vi "Dequeue.vi"(8 "error in (no error)":errorcluster, 10 "Dequeue Mode":T1, 11 "Messaging in":refnum<class "Messaging.lvclass">) -> (0 "error out":errorcluster, 1 "Data":variant, 2 "Message":string, 3 "Messaging out":refnum<class "Messaging.lvclass">)   [LabVIEW 2023, in "Messaging.lvclass"]
uses:
  Messaging.lvclass
  Messaging.lvclass/Messaging.ctl
  Msg/Msg.Q.DequeueMode.ctl
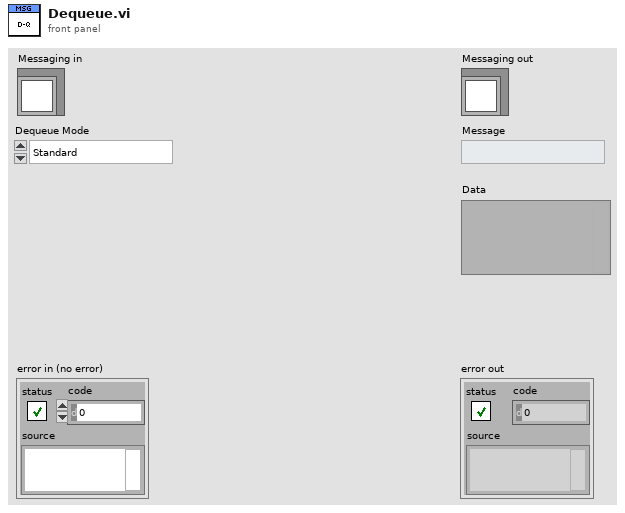
[diagram p1: front panel]
types:
  T1 = typedef "Msg.Q.DequeueMode.ctl" = enum16{"Standard", "Preview"}
  T2 = typedef "Msg.Q.Ref.ctl" = refnum<queue>
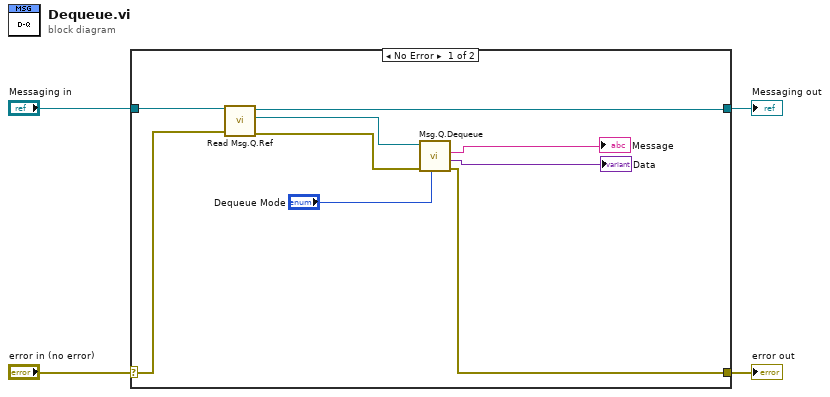
[diagram p0: block diagram]
diagram:
  n1 = case shown="No Error" "error in (no error)" {
    selector: "error in (no error)" -> [w12 w15]
    tunnel: [w5 w15] -> w3
    tunnel: [w11 w14] -> w1
    tunnel: "Messaging in" -> [w13 w14]
    frame No Error {
      n2 = call-dynamic "Read Msg.Q.Ref.vi"("error in (no error)"=w12, "Messaging in"=w13) -> ("error out"=w7:errorcluster, "Msg.Q.Ref"=w8:T2, "Messaging out"=w11:refnum<class "Messaging.lvclass">)  [unwired: 7 in]
      n3 = call "Msg.Q.Dequeue.vi"("Dequeue Mode"="Dequeue Mode", "Error (in)"=w7, "Msg.Q.Ref (in)"=w8) -> ("Error (out)"=w5:errorcluster, "Data"=→"Data":variant, "Message"=→"Message":string)  [unwired: 5 in, 1 out]
    }
    frame Error {
    }
  }
  "error out" <- w3
  "Messaging out" <- w1
